vi "log_error_to_file.vi"(11 "error_info":string[](array[string])) -> ()   [LabVIEW 2020]
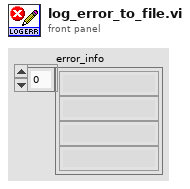
[diagram p1: front panel]
types:
  T1 = enum16{"open", "replace", "create", "open or create", "replace or create", "replace or create with confirmation"}
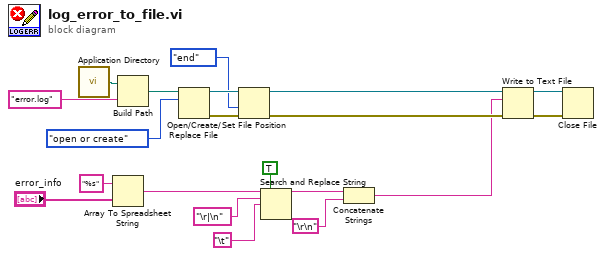
[diagram p0: block diagram]
diagram:
  n1 = call <vilib>:"Application Directory.vi"() -> ("Application Directory"=w13:path)
  n2 = Array To Spreadsheet String(array="error_info", 3:"%s" ("format string")) -> (spreadsheet string=w5:string)  [unwired: 1 in]
  n3 = Build Path(base path=w13, name or relative path="error.log") -> (appended path=w12:path)
  n4 = Open/Create/Replace File(file path (use dialog)=w12, operation (0:open)=T1."open or create") -> (refnum out=w18:refnum<file>, error out=w15:errorcluster)  [unwired: 4 in, 1 out]
  n5 = Set File Position(refnum=w18, from (0:start)=enum16{"start", "end", "current"}."end", error in=w15) -> (refnum out=w20:refnum<file>, error out=w16:errorcluster)  [unwired: 1 in]
  n6 = Search and Replace String(replace all?=TRUE ("Alle ersetzen? (F)"), input string=w5, search string="\r|\n" ("Such-String"), replace string="\t") -> (result string=w2:string)  [unwired: 4 in, 3 out]
  n7 = Concatenate Strings(w2, "\r\n") -> (w4:string)
  n8 = Write to Text File(file (use dialog)=w20, text=w4, error in=w16) -> (refnum out=w10:refnum<file>, error out=w9:errorcluster)  [unwired: 1 in, 1 out]
  n9 = Close File(refnum=w10, error in=w9) -> ()  [unwired: 2 out]
